vi "AlliGator Get Selected Plots and Reference Decay.vi"(8 "error in (no error)":errorcluster, 10 "Reference Decay":cluster{"t Array":dbl[], "I Array":dbl[]}, 11 "Selected Plot Info":T2) -> (0 "error out":errorcluster, 1 "Valid Reference Decay?":bool, 2 "Selected Plots":i32[](array[numeric]), 3 "XYGraph":T1, 4 "Reference Decay":cluster{"t Array":dbl[], "Value Array":dbl[]})   [LabVIEW 2021, in "AlliGator Decay Analysis.lvlib" / "AlliGator Decay Processing.lvlib"]
doc: "Get selected plot indices and reference decay."
uses:
  AlliGator Decay Processing.lvlib
  Graphs/XY Graph/XY Graph Selected Plot Info.ctl
  Graphs/XY Graph/XY Graph Refnum.ctl
  <vilib>/Utility/miscctls.llb/LVPoint32TypeDef.ctl
  AlliGator Decay Fit.lvlib
  Error/Error.lvlib
  Graphs/XY Graph/XY Graph Add-Ons.lvlib
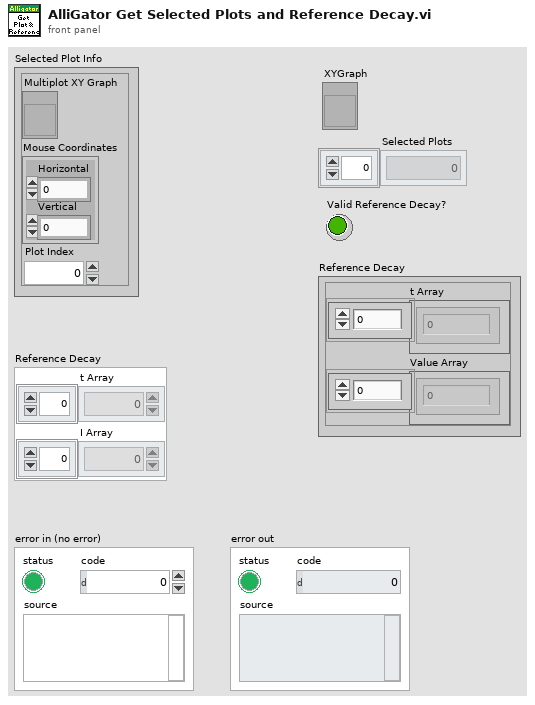
[diagram p1: front panel]
types:
  T1 = typedef "XY Graph Add-Ons.lvlib/XY Graph Refnum.ctl" = refnum<vi>
  T2 = typedef "XY Graph Add-Ons.lvlib/XY Graph Selected Plot Info.ctl" = cluster{"Multiplot XY Graph":T1, "Mouse Coordinates":T3, "Plot Index":i32}
  T3 = typedef "LVPoint32TypeDef.ctl" = cluster{"Horizontal":i32, "Vertical":i32}
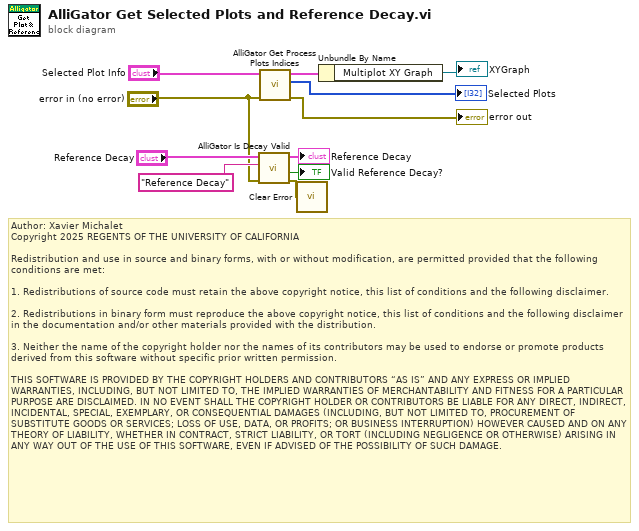
[diagram p0: block diagram]
diagram:
  # "Author: Xavier Michalet\nCopyright 2025 REGENTS OF THE UNIVERSITY OF CALIFORNIA\n\nRedistribution and use in source and binary forms, with or without modification, are permitted provided that the following conditions are met:\n\n1. Redistributions of source code must retain the above copyright notice, this list of conditions and the following disclaimer.\n\n2. Redistributions in binary form must reproduce the above copyright notice, this list of conditions and the following disclaimer in the documentation and/or other materials provided with the distribution.\n\n3. Neither the name of the copyright holder nor the names of its contributors may be used to endorse or promote products derived from this software without specific prior written permission.\n\nTHIS SOFTWARE IS PROVIDED BY THE COPYRIGHT HOLDERS AND CONTRIBUTORS “AS IS” AND ANY EXPRESS OR IMPLIED WARRANTIES, INCLUDING, BUT NOT LIMITED TO, THE IMPLIED WARRANTIES OF MERCHANTABILITY AND FITNESS FOR A PARTICULAR PURPOSE ARE DISCLAIMED. IN NO EVENT SHALL THE COPYRIGHT HOLDER OR CONTRIBUTORS BE LIABLE FOR ANY DIRECT, INDIRECT, INCIDENTAL, SPECIAL, EXEMPLARY, OR CONSEQUENTIAL DAMAGES (INCLUDING, BUT NOT LIMITED TO, PROCUREMENT OF SUBSTITUTE GOODS OR SERVICES; LOSS OF USE, DATA, OR PROFITS; OR BUSINESS INTERRUPTION) HOWEVER CAUSED AND ON ANY THEORY OF LIABILITY, WHETHER IN CONTRACT, STRICT LIABILITY, OR TORT (INCLUDING NEGLIGENCE OR OTHERWISE) ARISING IN ANY WAY OUT OF THE USE OF THIS SOFTWARE, EVEN IF ADVISED OF THE POSSIBILITY OF SUCH DAMAGE."
  n1 = call "AlliGator Is Decay Valid.vi"("Error In"="error in (no error)", "Plot Name"="Reference Decay", "Decay"="Reference Decay") -> ("Error Out"=w7:errorcluster, "Is Valid?"=→"Valid Reference Decay?":bool, "Decay (dup)"=→"Reference Decay":cluster{"t Array":dbl[], "Value Array":dbl[]})  [unwired: 5 in, 1 out]
  n2 = call "AlliGator Get Process Plots Indices.vi"("error in (no error)"="error in (no error)", "Selected Plot Info"="Selected Plot Info") -> ("error out"=→"error out":errorcluster, "Selected Plots"=→"Selected Plots":i32[], "Selected Plot Info (dup)"=w6:T2)  [unwired: 7 in]
  n3 = call "Clear Error.vi"("Error In"=w7) -> ()  [unwired: 8 in, 1 out]
  n4 = Unbundle By Name(w6) -> ("Multiplot XY Graph"=→"XYGraph":T1)
